vi "Remove Sensor Asic.vi"(8 "error in (no error)":errorcluster caption="错误输入（无错误）", 10 "asicHandle":i32, 11 "sensorHandle":i32) -> (0 "error out":errorcluster caption="错误输出", 2 "asicHandleout":i32, 3 "SensorHandleout":i32)   [LabVIEW 2018]
doc: "extern int __stdcall APSxRemoveSensorAsic (int sensorHandle, IN int asicHandle);"
uses:
  APSx.dll/APSx.dll
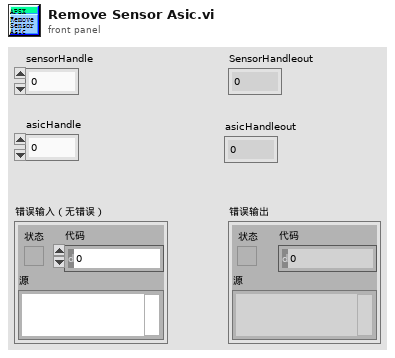
[diagram p1: front panel]
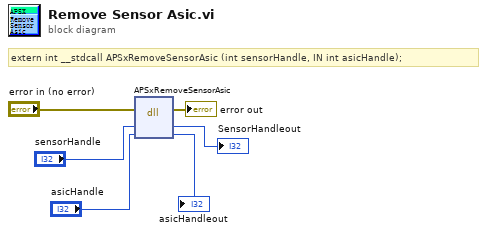
[diagram p0: block diagram]
diagram:
  # "extern int __stdcall APSxRemoveSensorAsic (int sensorHandle, IN int asicHandle);"
  n1 = dll-call lib="PTH2[abs D项目Feng恒隆项目Labview传感器对中台SourcesAPSx.dllAPSx.*" fn="APSxRemoveSensorAsic"(error in="error in (no error)", "sensorHandle"="sensorHandle", "asicHandle"="asicHandle") -> (error out=→"error out":errorcluster, "sensorHandle"=→"SensorHandleout":i32, "asicHandle"=→"asicHandleout":i32)  [unwired: 3 in, 1 out]
